vi "Webcam.vi"(8 "error in (no error)":errorcluster, 10 "Image Name":string="webcam", 11 "Session In":T2="cam0") -> (0 "error out":errorcluster, 3 "Image":T1(plugin-control))   [LabVIEW 2014]
uses:
  <vilib>/userdefined/High Color/IMAQdx.ctl
  <vilib>/vision/driver/NI_Vision_Acquisition_Software.lvlib
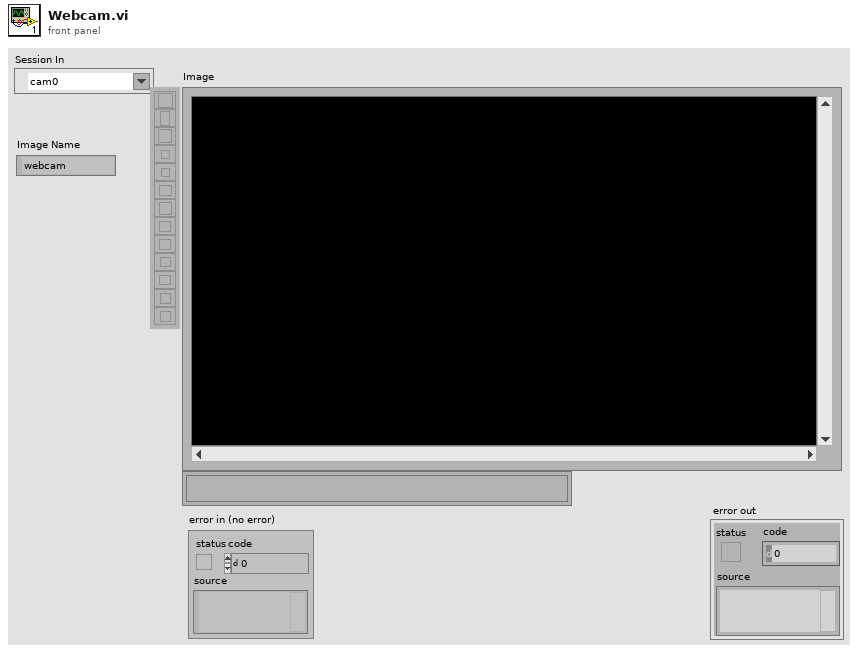
[diagram p1: front panel]
types:
  T1 = typedef "IMAQ Image.ctl" = refnum<image>
  T2 = typedef "IMAQdx.ctl" = refnum<k21>
  T3 = typedef "Image Type" = u32
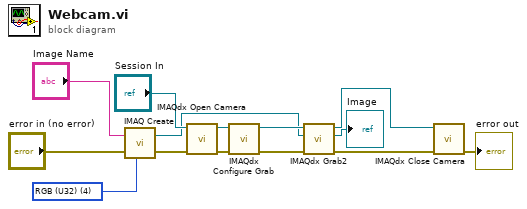
[diagram p0: block diagram]
diagram:
  w7 = T3 4 items=["Grayscale (U8)", "Grayscale (I16)", "Grayscale (SGL)", "Complex (CSG)", "RGB (U32)", "HSL (U32)", "RGB (U64)", "Grayscale (U16)"] ("Image Type")
  n1 = call "IMAQ Create"("Image Name"="Image Name", "Image Type"=w7, "error in (no error)"="error in (no error)") -> ("New Image"=w6:T1, "error out"=w4:errorcluster)  [unwired: 2 in]
  n2 = call <vilib>:"IMAQdx Open Camera.vi"("error in"=w4, "Session In"="Session In") -> ("error out"=w10:errorcluster, "Session Out"=w11:T2)  [unwired: 8 in]
  n3 = call <vilib>:"IMAQdx Configure Grab.vi"("error in"=w10, "Session In"=w11) -> ("error out"=w12:errorcluster, "Session Out"=w13:T2)  [unwired: 8 in]
  n4 = call <vilib>:"IMAQdx Grab2.vi"("error in"=w12, "Image In"=w6, "Session In"=w13) -> ("error out"=w14:errorcluster, "Image Out"=→"Image":T1, "Session Out"=w8:T2)  [unwired: 5 in, 1 out]
  n5 = call <vilib>:"IMAQdx Close Camera.vi"("error in"=w14, "Session In"=w8) -> ("error out"=→"error out":errorcluster)  [unwired: 9 in]
